vi "Input Quantities.vi"() -> ()   [LabVIEW 2013]
uses:
  qwtblvlib/TD Quantity.ctl
  <vilib>/Analysis/Matrix/Datatypes/RealMatrix.ctl
  globals.vi
  <vilib>/Utility/xml.llb/Write to XML File(string).vi
  <vilib>/Utility/xml.llb/Read From XML File(string).vi
  <vilib>/Utility/file.llb/Read From Spreadsheet File (DBL).vi
  <vilib>/Analysis/Matrix/Numeric/Conversions/Matrix To Array - RM.vi
  <vilib>/Analysis/Matrix/NI_Matrix.lvlib
  qwtblvlib/QWTBLVLib.lvlib
panel:
  out "current Q index":i32 min=0
  in  "r-randomize":bool
  in  "corr-default":bool
  in  "dof-fill":bool
  in  "uncertainty-fill":bool
  in  "value-load CSV":bool
  in  "hide this panel":bool
  in  "load 2clmn csv":bool
  in  "generate wvfrm":bool
  in  "Q changed signal":bool
  in  "reload Q list signal":bool
  in  "reload Q signal":bool
  in  "Q":T1={"Name"="", "Value"=[[1.0]], "Uncertainty"=[[1.0]], "Degrees of Freedom"=[[10.0]], "Correlation"=[[10.0]], "Randomized uncertainty"=[[10.0]]} caption="Selected Quantity"
  in  "load Q":bool
  in  "save Q":bool
  in  "Q list":i32(listbox) caption="List of\nInput Quantities"
  in  "remove Q":bool
  in  "add Q":bool
  in  "rand-clear":bool
  in  "corr-clear":bool
  in  "dof-clear":bool
  in  "uncertainty-clear":bool
  in  "value-clear":bool
  # "Input Quantities"
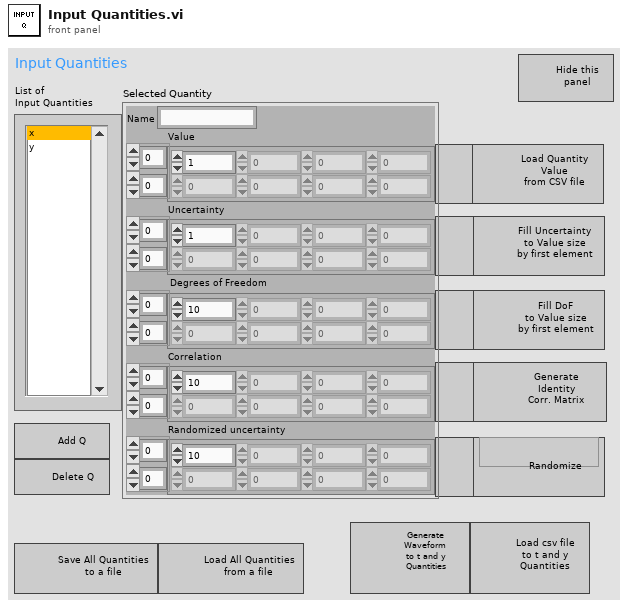
[diagram p1: front panel]
types:
  T1 = typedef "QWTBLVLib.lvlib/TD Quantity.ctl" = cluster{"Name":string, "Value":dbl[][], "Uncertainty":dbl[][], "Degrees of Freedom":dbl[][], "Correlation":dbl[][], "Randomized uncertainty":dbl[][]}
  T2 = enum32{"Invalid", "Standard", "Closed", "Hidden", "Minimized", "Maximized"}
  T3 = cluster{"Name":string, "Value":dbl[][], "Uncertainty":dbl[][], "Degrees of\nFreedom":dbl[][], "Correlation":dbl[][], "Randomized uncertainty":dbl[][]}
  T4 = typedef "NI_Matrix.lvlib/RealMatrix.ctl" = dbl[][]
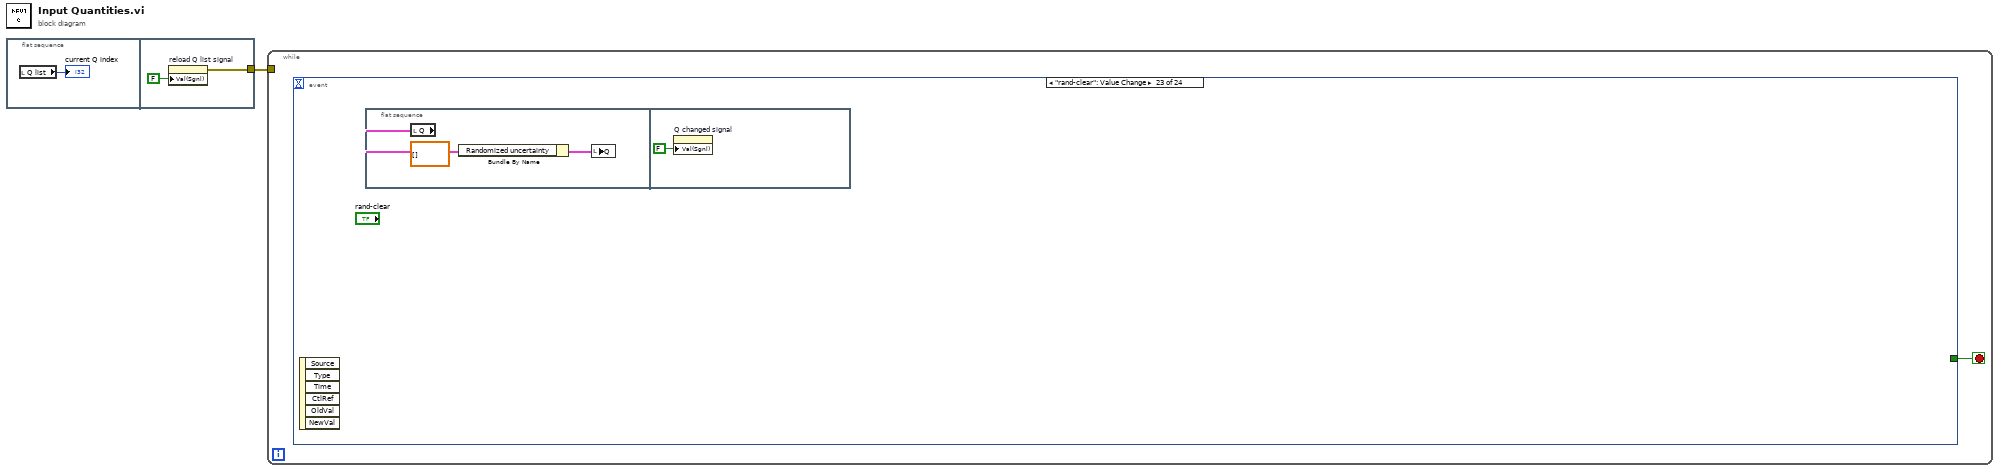
[diagram p0: block diagram]
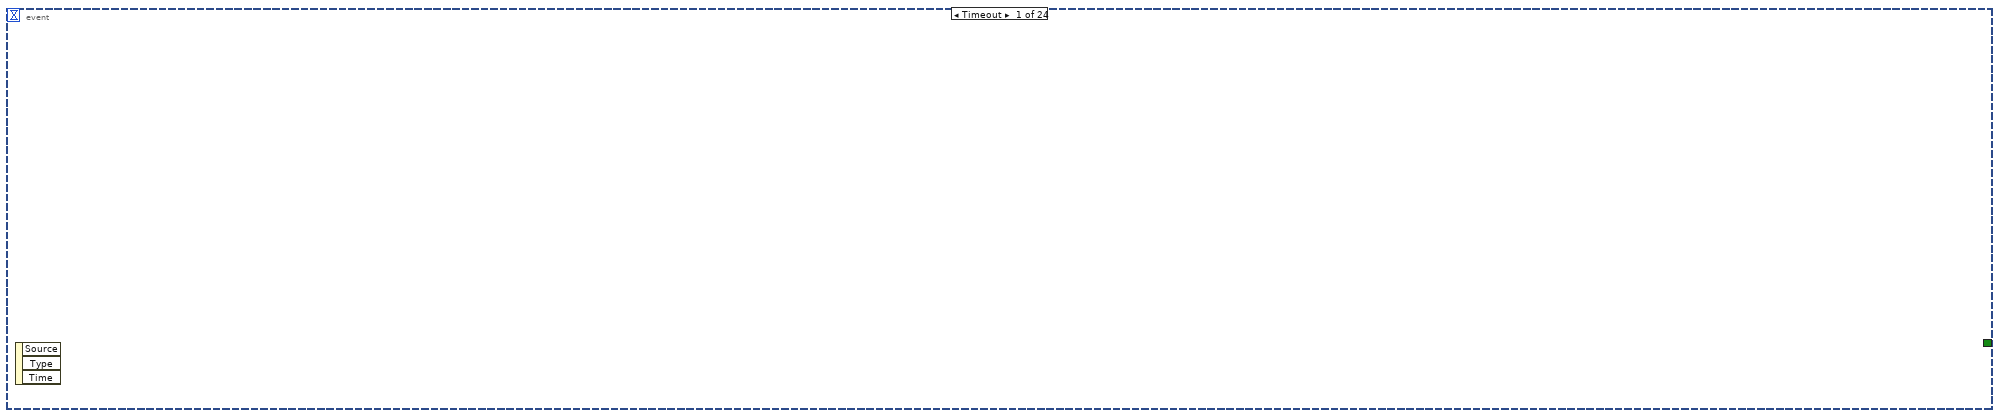
[diagram p2: hidden frame]
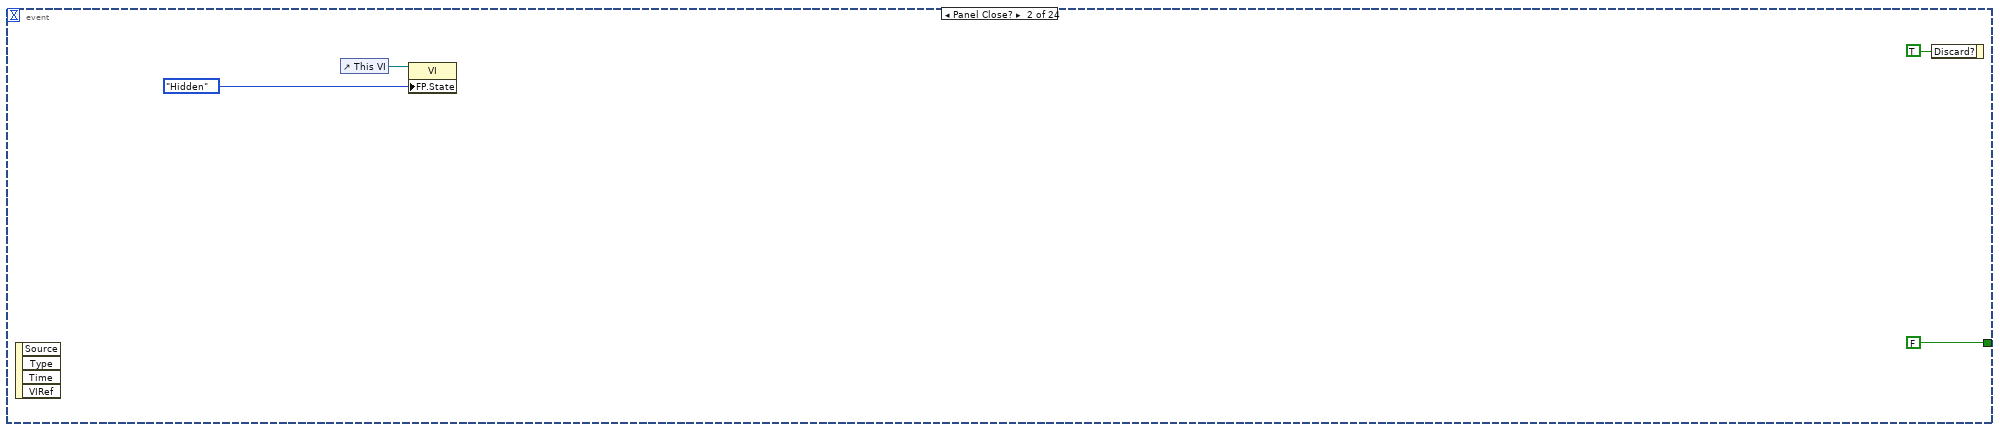
[diagram p3: hidden frame]
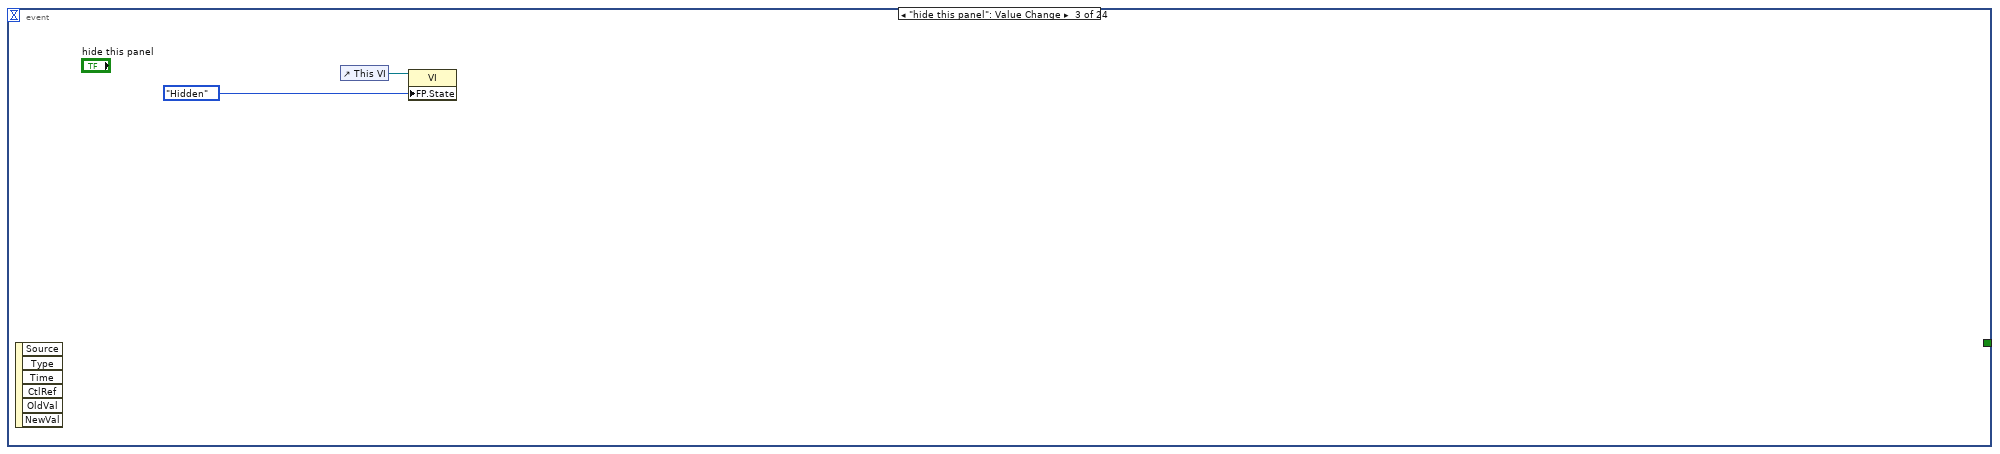
[diagram p4: hidden frame]
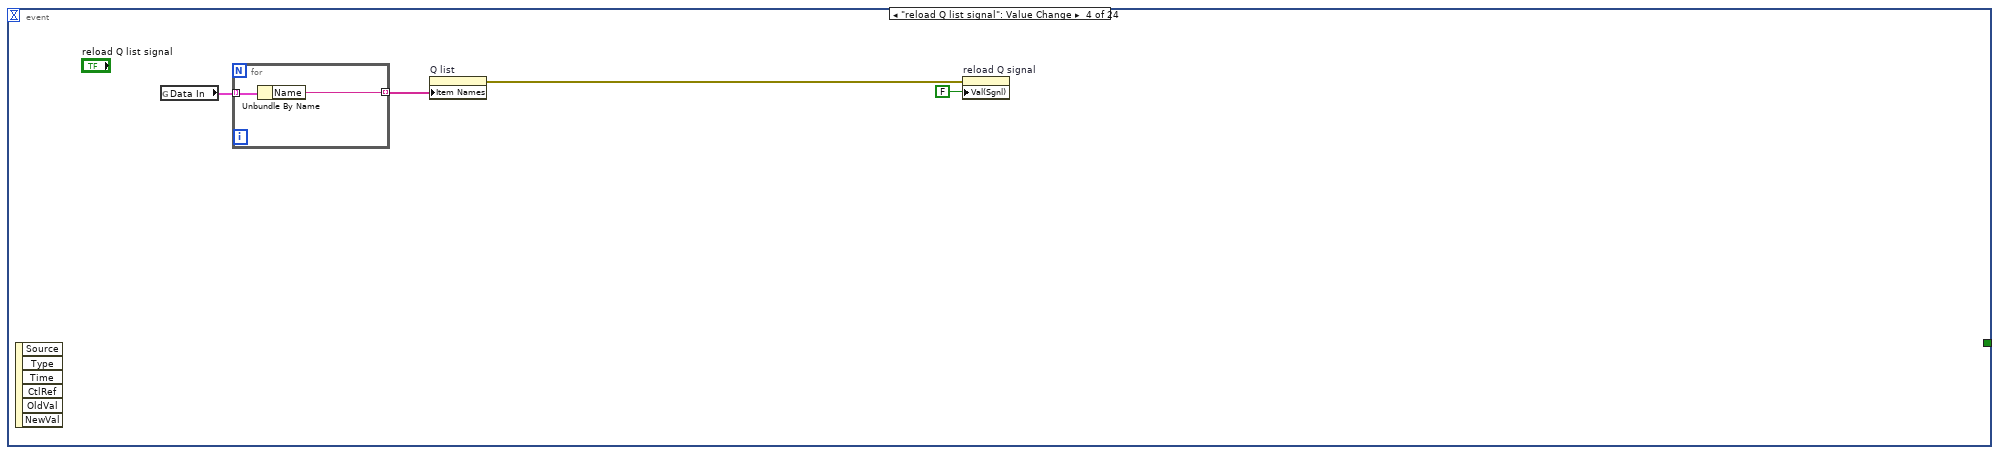
[diagram p5: hidden frame]
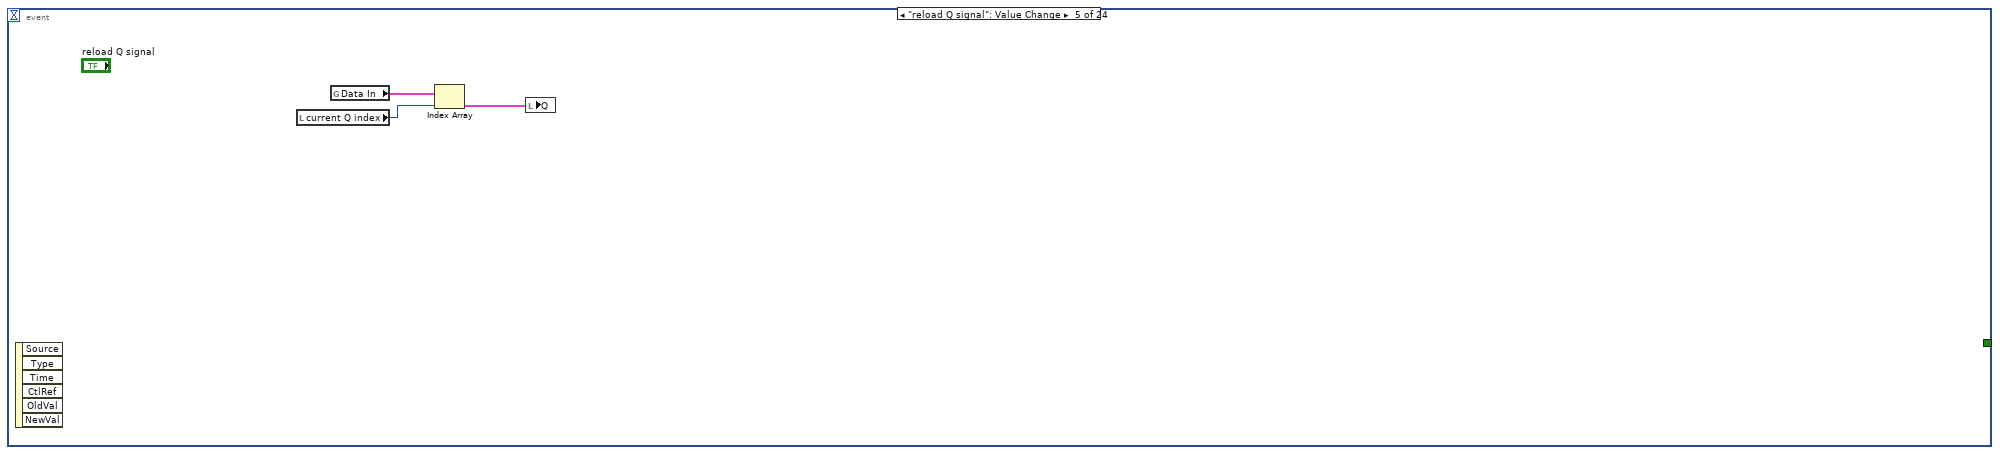
[diagram p6: hidden frame]
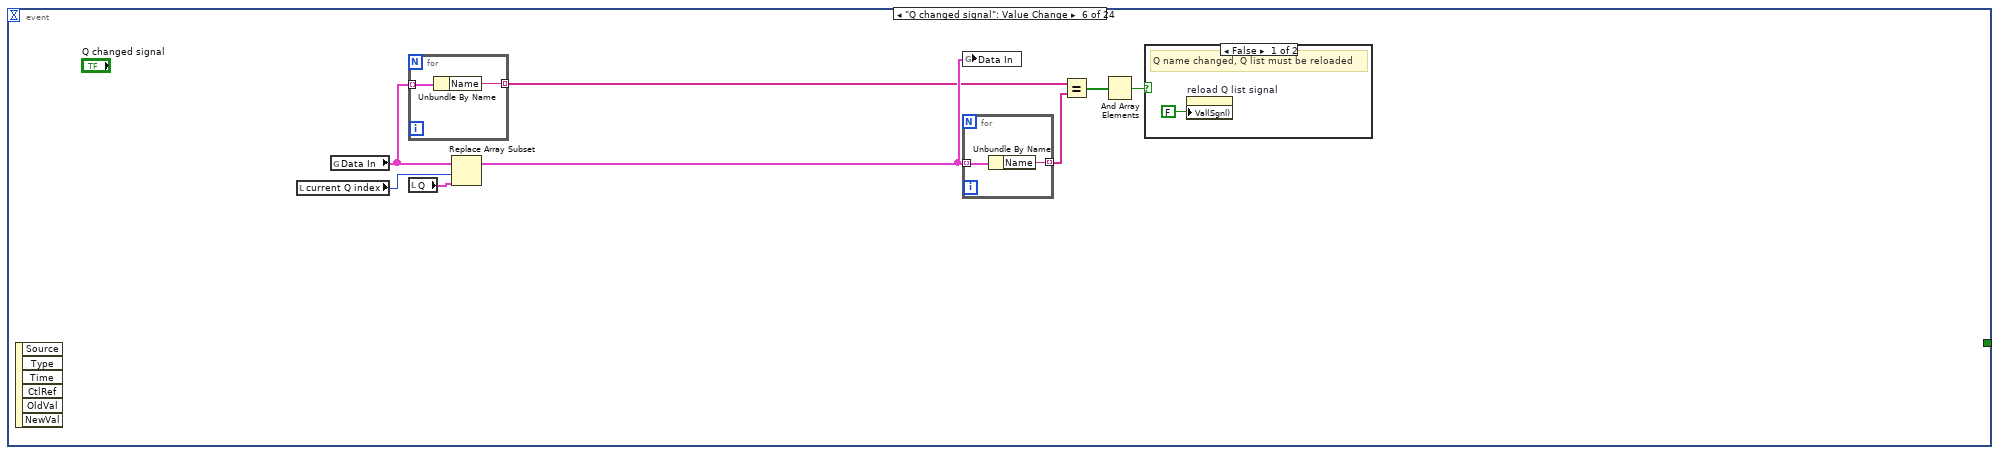
[diagram p7: hidden frame]
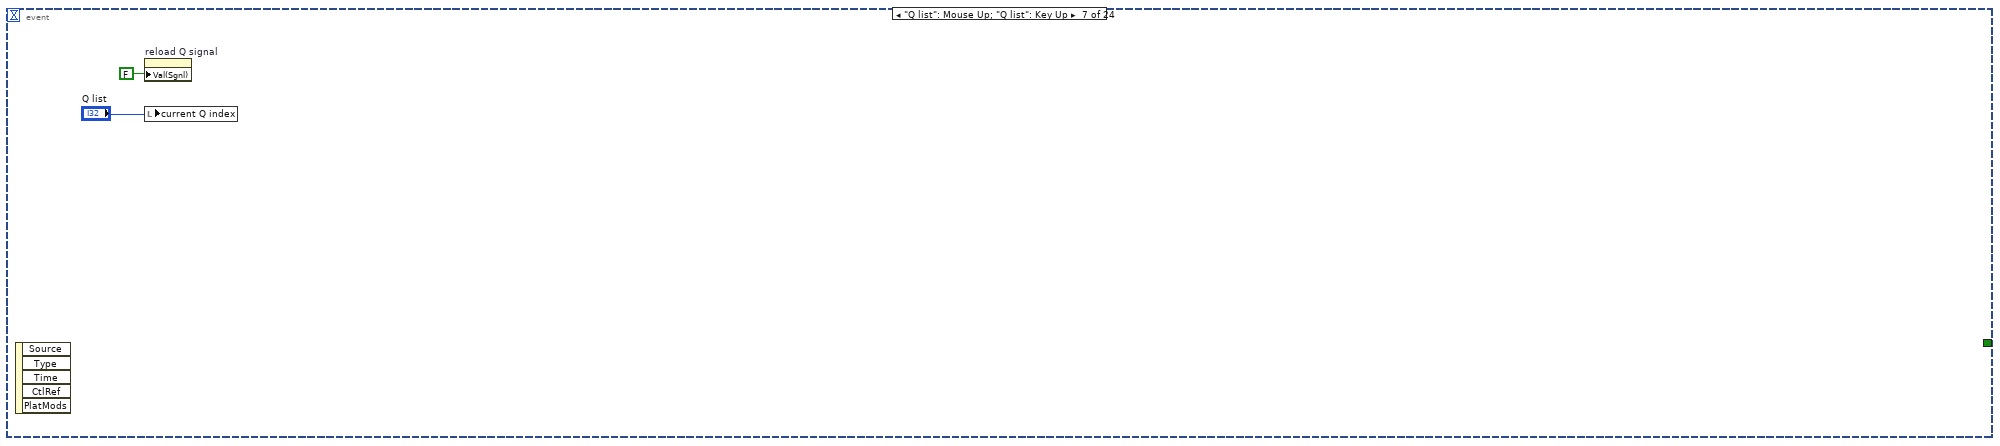
[diagram p9: hidden frame]
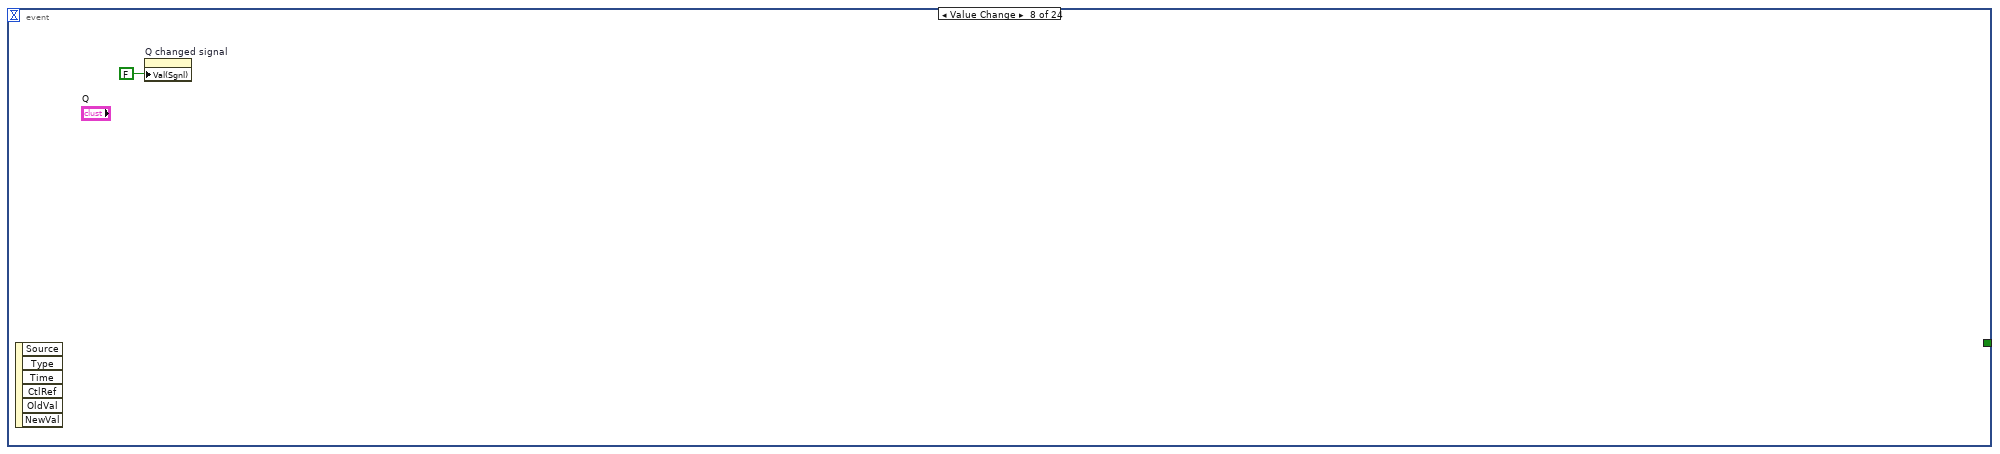
[diagram p10: hidden frame]
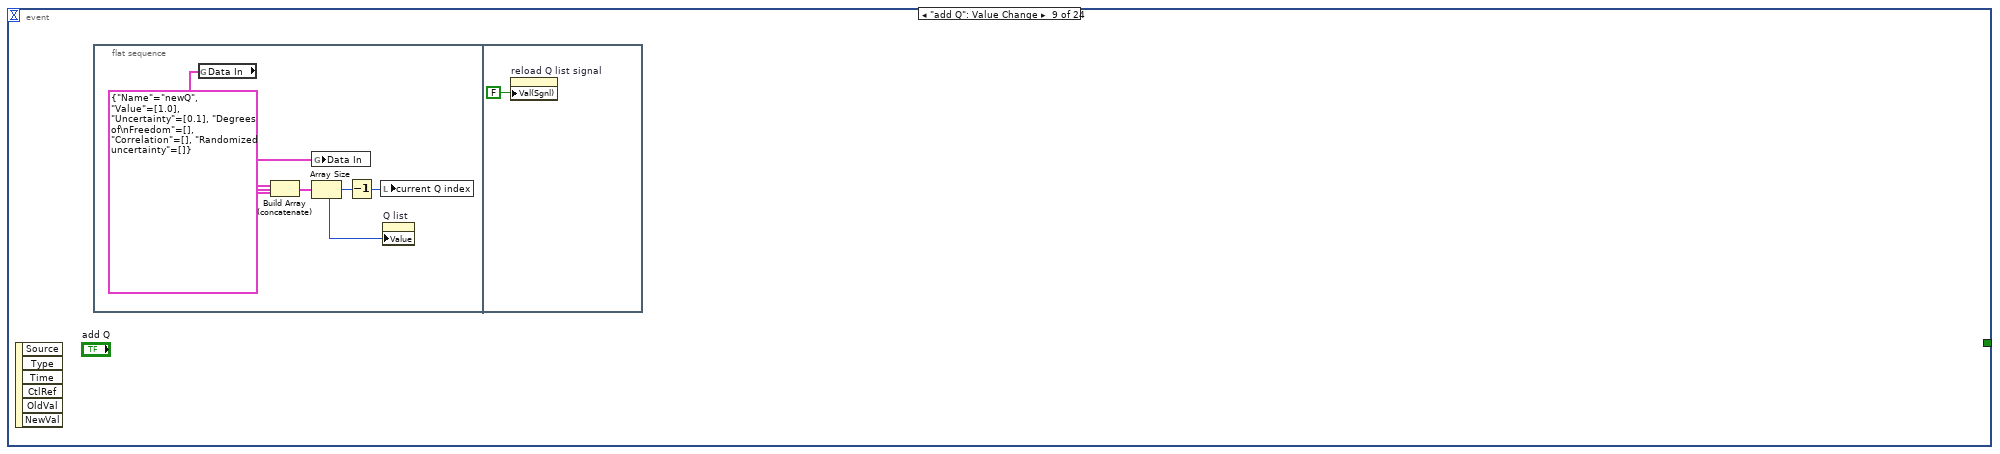
[diagram p11: hidden frame]
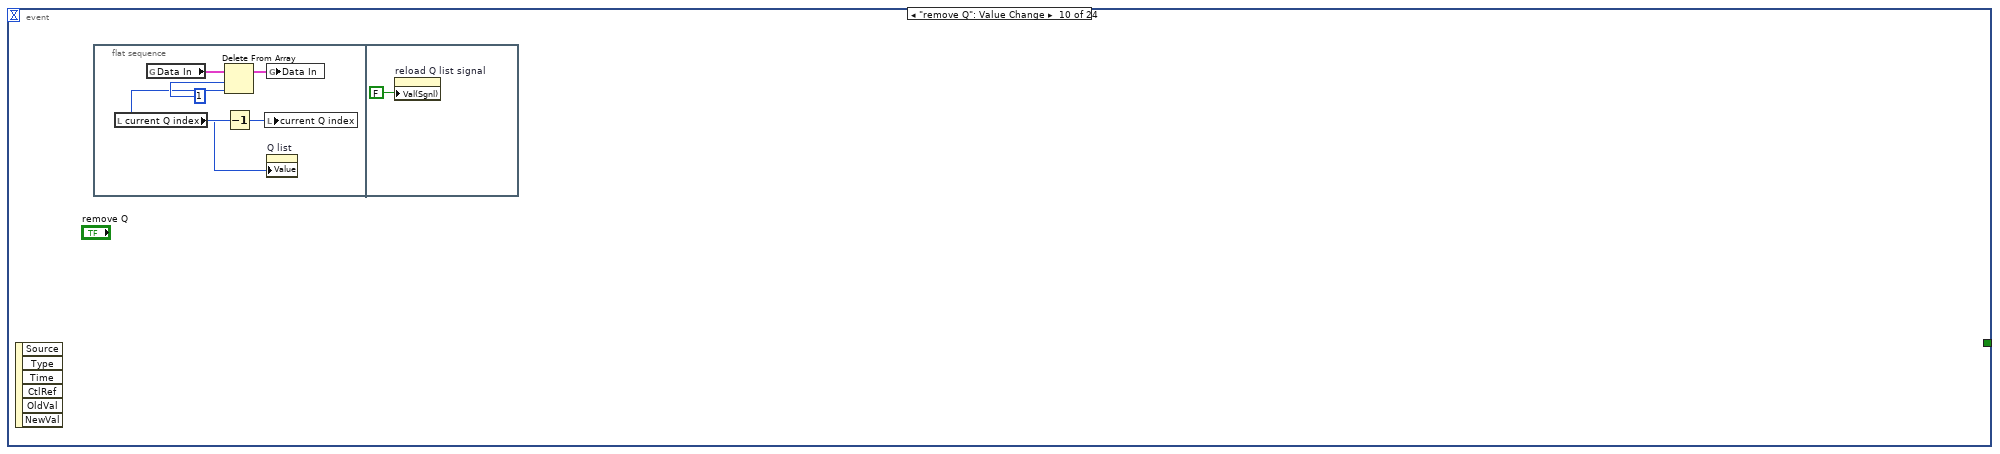
[diagram p12: hidden frame]
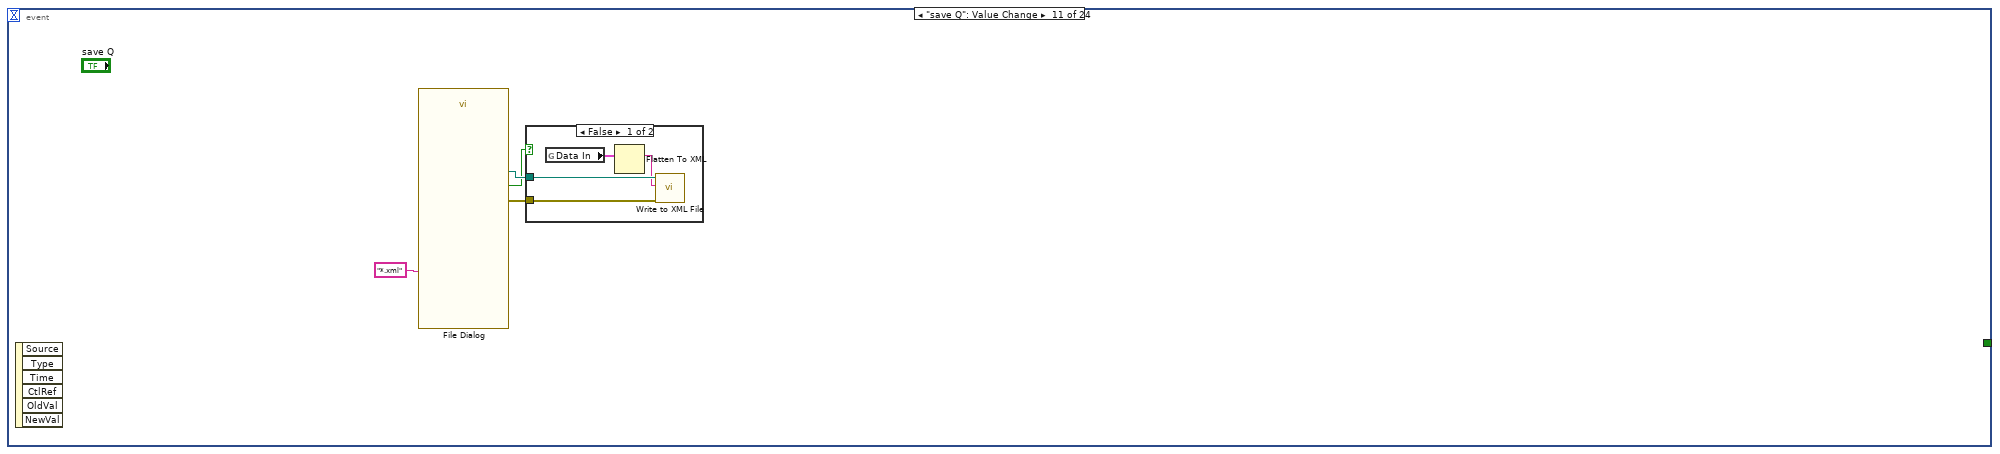
[diagram p13: hidden frame]
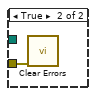
[diagram p14: hidden frame]
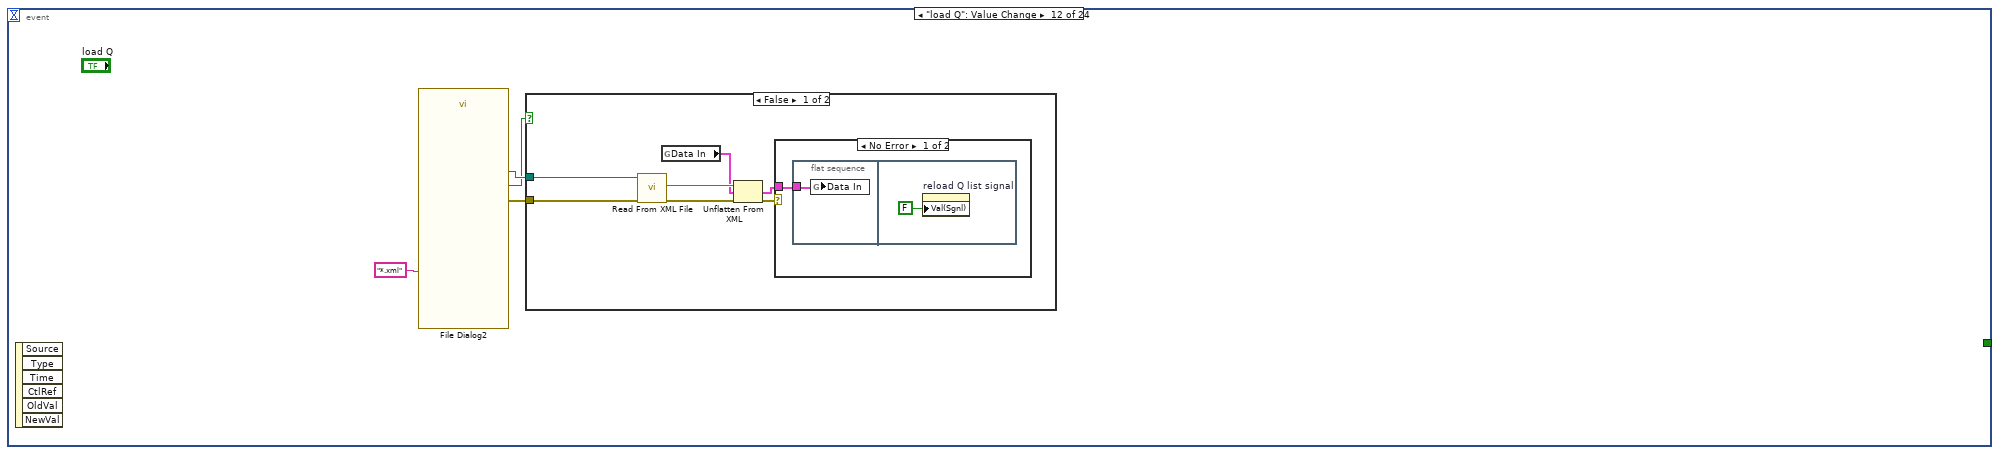
[diagram p15: hidden frame]
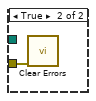
[diagram p17: hidden frame]
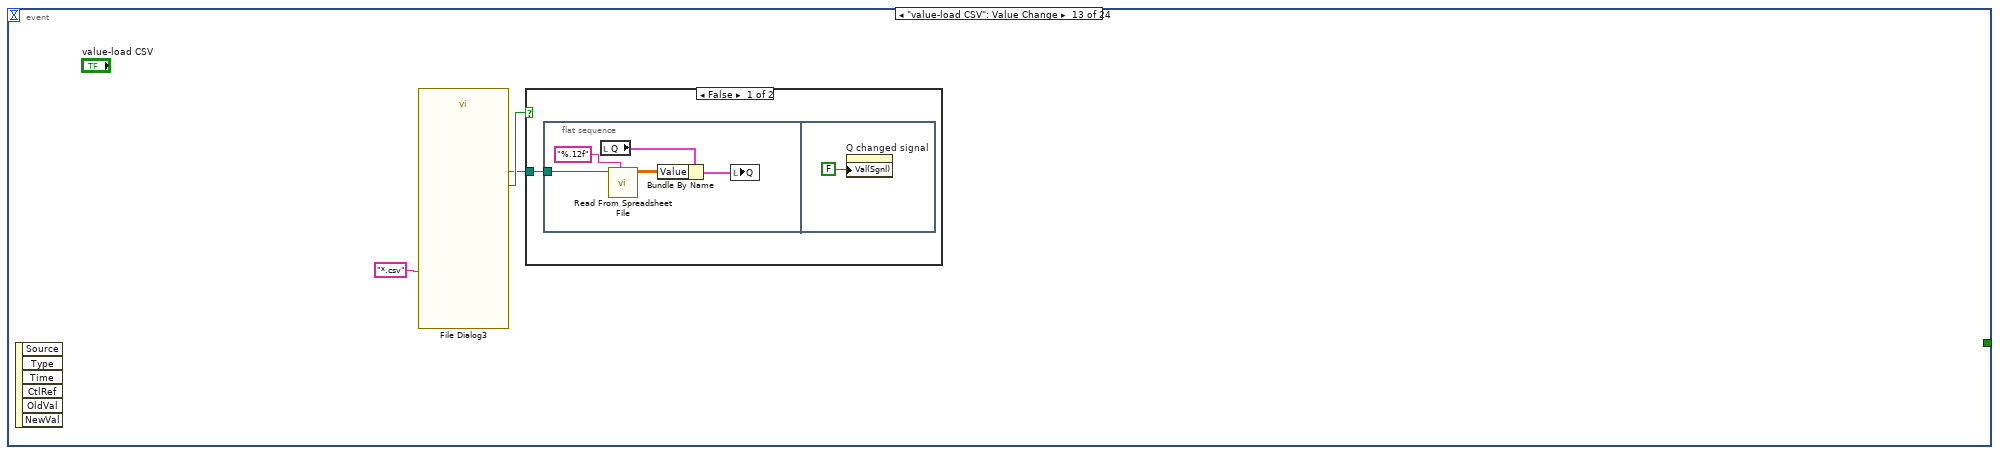
[diagram p18: hidden frame]
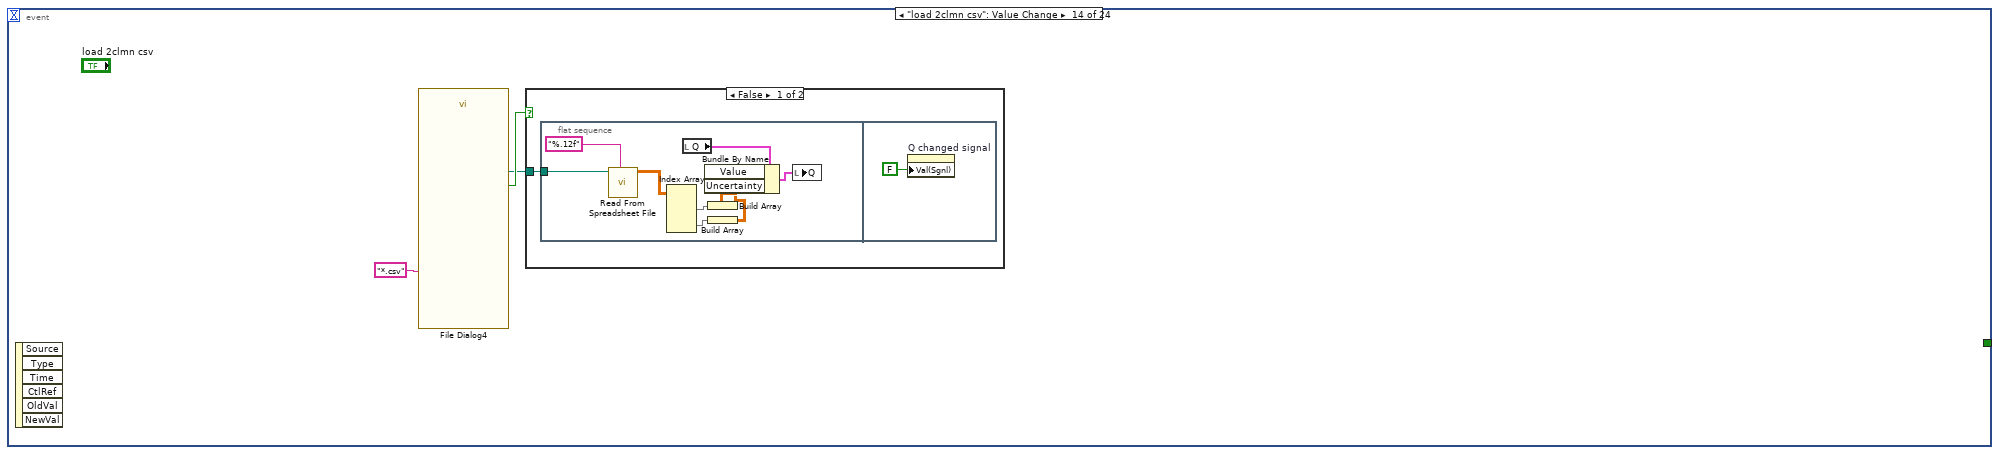
[diagram p20: hidden frame]
diagram:
  n1 = flat-sequence {
    tunnel: [w3] -> w1
    frame #0 {
      n2 = local read "Q list"() -> (→"current Q index":i32)
    }
    frame #1 {
      n3 = property on="reload Q list signal" class="Bool (strict)"("Val(Sgnl)"=FALSE ("Value (Signaling)")) -> (error out=w3:errorcluster)  [unwired: 2 in, 1 out]
    }
  }
  n4 = while {
    tunnel: w1 -> [_]
    stop <- w5 stop-if-true
    n5 = event shown="[22] \"rand-clear\": Value Change" {
      selector: _ -> [_ _ _ _ _ _ _ _ _ _ _ _ _ _ _ _ _ _ _ _ _ _ _ _]
      dyn-events: _ -> [_ _ _ _ _ _ _ _ _ _ _ _ _ _ _ _ _ _ _ _ _ _ _ _]
      timeout: _ -> [_ _ _ _ _ _ _ _ _ _ _ _ _ _ _ _ _ _ _ _ _ _ _ _]
      tunnel: [_ FALSE _ _ _ _ _ _ _ _ _ _ _ _ _ _ _ _ _ _ _ _ _ _] -> w5
      event Timeout {
        n6 = event-data() -> ()  [unwired: 1 in, 3 out]
      }
      event Panel Close? {
        n7 = event-data() -> ()  [unwired: 1 in, 4 out]
        n8 = control-ref of="This VI"() -> (w7:refnum<vi>)
        n9 = property class="VI"(reference=w7, "FP.State"=T2."Hidden" ("Front Panel Window:State")) -> ()  [unwired: 1 in, 2 out]
        n10 = event-data("Discard?"=TRUE) -> ()  [unwired: 1 in, 1 out]
      }
      event "hide this panel": Value Change {
        n11 = event-data() -> ()  [unwired: 1 in, 6 out]
        n12 = control-ref of="This VI"() -> (w11:refnum<vi>)
        n13 = property class="VI"(reference=w11, "FP.State"=T2."Hidden" ("Front Panel Window:State")) -> ()  [unwired: 1 in, 2 out]
      }
      event "reload Q list signal": Value Change {
        n14 = event-data() -> ()  [unwired: 1 in, 6 out]
        n15 = global read "globals.vi" "Data In"() -> (w14:T1[])
        n16 = for {
          tunnel: [w17] -> w13 mode=indexing
          tunnel: w14 -> [w16] mode=indexing
          n17 = Unbundle By Name(w16) -> ("Name"=w17:string)
        }
        n18 = property on="Q list" class="LstBox (strict)"("Item Names"=w13) -> (error out=w12:errorcluster)  [unwired: 2 in, 1 out]
        n19 = property on="reload Q signal" class="Bool (strict)"(error in=w12, "Val(Sgnl)"=FALSE ("Value (Signaling)")) -> ()  [unwired: 1 in, 2 out]
      }
      event "reload Q signal": Value Change {
        n20 = event-data() -> ()  [unwired: 1 in, 6 out]
        n21 = local read "current Q index"() -> (w18:i32)
        n22 = global read "globals.vi" "Data In"() -> (w20:T1[])
        n23 = Index Array(array=w20, index=w18) -> (element=w19:T1)
        n24 = local write "Q"(w19) -> ()
      }
      event "Q changed signal": Value Change {
        n25 = event-data() -> ()  [unwired: 1 in, 6 out]
        n26 = local read "current Q index"() -> (w21:i32)
        n27 = global read "globals.vi" "Data In"() -> (w27:T1[])
        n28 = for {
          tunnel: [w32] -> w25 mode=indexing
          tunnel: w27 -> [w31] mode=indexing
          n29 = Unbundle By Name(w31) -> ("Name"=w32:string)
        }
        n30 = local read "Q"() -> (w28:T1)
        n31 = Replace Array Subset(array=w27, new element=w28, index=w21) -> (w26:T1[])
        n32 = global write "globals.vi" "Data In"(w26) -> ()
        n33 = for {
          tunnel: [w30] -> w23 mode=indexing
          tunnel: w26 -> [w29] mode=indexing
          n34 = Unbundle By Name(w29) -> ("Name"=w30:string)
        }
        n35 = Equal?(x=w25, y=w23) -> (x = y?=w22:bool[])
        n36 = And Array Elements(Boolean array=w22) -> (logical AND=w24:bool)
        n37 = case shown="False" w24 {
          frame False {
            # "Q name changed, Q list must be reloaded"
            n38 = property on="reload Q list signal" class="Bool (strict)"("Val(Sgnl)"=FALSE ("Value (Signaling)")) -> ()  [unwired: 2 in, 2 out]
          }
          frame True {
          }
        }
      }
      event "Q list": Mouse Up; "Q list": Key Up {
        n39 = event-data() -> ()  [unwired: 1 in, 5 out]
        n40 = property on="reload Q signal" class="Bool (strict)"("Val(Sgnl)"=FALSE ("Value (Signaling)")) -> ()  [unwired: 2 in, 2 out]
        n41 = local write "current Q index"("Q list") -> ()
      }
      event Value Change {
        n42 = event-data() -> ()  [unwired: 1 in, 6 out]
        n43 = property on="Q changed signal" class="Bool (strict)"("Val(Sgnl)"=FALSE ("Value (Signaling)")) -> ()  [unwired: 2 in, 2 out]
      }
      event "add Q": Value Change {
        n44 = event-data() -> ()  [unwired: 1 in, 6 out]
        n45 = flat-sequence {
          frame #0 {
            n46 = global read "globals.vi" "Data In"() -> (w39:T1[])
            n47 = Build Array (concatenate)(w39, T3 {"Name"="newQ", "Value"=[[1.0]], "Uncertainty"=[[0.1]], "Degrees of\nFreedom"=[], "Correlation"=[], "Randomized uncertainty"=[]} ("Quantity")) -> (w38:T1[])
            n48 = global write "globals.vi" "Data In"(w38) -> ()
            n49 = Array Size(array=w38) -> (size(s)=w41:i32)
            n50 = Decrement(x=w41) -> (x-1=w37:i32)
            n51 = local write "current Q index"(w37) -> ()
            n52 = property on="Q list" class="LstBox (strict)"("Value"=w37) -> ()  [unwired: 2 in, 2 out]
          }
          frame #1 {
            n53 = property on="reload Q list signal" class="Bool (strict)"("Val(Sgnl)"=FALSE ("Value (Signaling)")) -> ()  [unwired: 2 in, 2 out]
          }
        }
      }
      event "remove Q": Value Change {
        n54 = event-data() -> ()  [unwired: 1 in, 6 out]
        n55 = flat-sequence {
          frame #0 {
            n56 = local read "current Q index"() -> (w44:i32)
            n57 = global read "globals.vi" "Data In"() -> (w46:T1[])
            n58 = Delete From Array(array=w46, length=1, index=w44) -> (array with subset deleted=w45:T1[])  [unwired: 1 out]
            n59 = Decrement(x=w44) -> (x-1=w43:i32)
            n60 = local write "current Q index"(w43) -> ()
            n61 = global write "globals.vi" "Data In"(w45) -> ()
            n62 = property on="Q list" class="LstBox (strict)"("Value"=w43) -> ()  [unwired: 2 in, 2 out]
          }
          frame #1 {
            n63 = property on="reload Q list signal" class="Bool (strict)"("Val(Sgnl)"=FALSE ("Value (Signaling)")) -> ()  [unwired: 2 in, 2 out]
          }
        }
      }
      event "save Q": Value Change {
        n64 = event-data() -> ()  [unwired: 1 in, 6 out]
        n65 = call "File Dialog"("pattern (all files)"="*.xml") -> ("selected path"=w52:path, "cancelled"=w50:bool, "error out"=w51:errorcluster)  [unwired: 11 in, 1 out]
        n66 = case shown="False" w50 {
          tunnel: w51 -> [w55 w57]
          tunnel: w52 -> [w56 _]
          frame False {
            n67 = global read "globals.vi" "Data In"() -> (w53:T1[])
            n68 = Flatten To XML(anything=w53) -> (xml string=w54:string)
            n69 = call-poly <vilib>:"Write to XML File.vi"("error in (no error)"=w55, "XML Input"=w54, "XML File Path"=w56) -> ()  [unwired: 6 in, 3 out]
          }
          frame True {
            n70 = call <vilib>:"Clear Errors.vi"("error in (no error)"=w57) -> ()  [unwired: 6 in, 1 out]
          }
        }
      }
      event "load Q": Value Change {
        n71 = event-data() -> ()  [unwired: 1 in, 6 out]
        n72 = call "File Dialog2"("pattern (all files)"="*.xml") -> ("selected path"=w61:path, "cancelled"=w59:bool, "error out"=w60:errorcluster)  [unwired: 11 in, 1 out]
        n73 = case shown="False" w59 {
          tunnel: w60 -> [w67 w72]
          tunnel: w61 -> [w68 _]
          frame False {
            n74 = call-poly <vilib>:"Read From XML File.vi"("error in (no error)"=w67, "XML File Path"=w68) -> ("error out"=w65:errorcluster, "XML Elements"=w66:string)  [unwired: 7 in, 1 out]
            n75 = global read "globals.vi" "Data In"() -> (w62:T1[])
            n76 = Unflatten From XML(xml string=w66, type=w62, error in (no error)=w65) -> (value=w63:T1[], error out=w64:errorcluster)
            n77 = case shown="No Error" w64 {
              tunnel: w63 -> [w69 _]
              frame No Error {
                n78 = flat-sequence {
                  tunnel: w69 -> [w70]
                  frame #0 {
                    n79 = global write "globals.vi" "Data In"(w70) -> ()
                  }
                  frame #1 {
                    n80 = property on="reload Q list signal" class="Bool (strict)"("Val(Sgnl)"=FALSE ("Value (Signaling)")) -> ()  [unwired: 2 in, 2 out]
                  }
                }
              }
              frame Error {
              }
            }
          }
          frame True {
            n81 = call <vilib>:"Clear Errors.vi"("error in (no error)"=w72) -> ()  [unwired: 6 in, 1 out]
          }
        }
      }
      event "value-load CSV": Value Change {
        n82 = event-data() -> ()  [unwired: 1 in, 6 out]
        n83 = call "File Dialog3"("pattern (all files)"="*.csv") -> ("selected path"=w73:path, "cancelled"=w74:bool)  [unwired: 11 in, 2 out]
        n84 = case shown="False" w74 {
          tunnel: w73 -> [w76 _]
          frame False {
            n85 = flat-sequence {
              tunnel: w76 -> [w81]
              frame #0 {
                n86 = local read "Q"() -> (w80:T1)
                n87 = call-poly <vilib>:"Read From Spreadsheet File.vi"("format (%.3f)"="%.12f", "file path (dialog if empty)"=w81) -> ("all rows"=w79:dbl[][])  [unwired: 5 in, 4 out]
                n88 = Bundle By Name(cluster=w80, "Value"=w79) -> (w78:T1)
                n89 = local write "Q"(w78) -> ()
              }
              frame #1 {
                n90 = property on="Q changed signal" class="Bool (strict)"("Val(Sgnl)"=FALSE ("Value (Signaling)")) -> ()  [unwired: 2 in, 2 out]
              }
            }
          }
          frame True {
          }
        }
      }
      event "load 2clmn csv": Value Change {
        n91 = event-data() -> ()  [unwired: 1 in, 6 out]
        n92 = call "File Dialog4"("pattern (all files)"="*.csv") -> ("selected path"=w83:path, "cancelled"=w84:bool)  [unwired: 11 in, 2 out]
        n93 = case shown="False" w84 {
          tunnel: w83 -> [w86 _]
          frame False {
            n94 = flat-sequence {
              tunnel: w86 -> [w95]
              frame #0 {
                n95 = call-poly <vilib>:"Read From Spreadsheet File.vi"("format (%.3f)"="%.12f", "file path (dialog if empty)"=w95) -> ("all rows"=w91:dbl[][])  [unwired: 5 in, 4 out]
                n96 = Index Array(array=w91) -> (element #1=w90:dbl[], element #2=w87:dbl[])  [unwired: 4 in]
                n97 = local read "Q"() -> (w94:T1)
                n98 = Build Array(w90) -> (w89:dbl[][])
                n99 = Build Array(w87) -> (w88:dbl[][])
                n100 = Bundle By Name(cluster=w94, "Value"=w89, "Uncertainty"=w88) -> (w93:T1)
                n101 = local write "Q"(w93) -> ()
              }
              frame #1 {
                n102 = property on="Q changed signal" class="Bool (strict)"("Val(Sgnl)"=FALSE ("Value (Signaling)")) -> ()  [unwired: 2 in, 2 out]
              }
            }
          }
          frame True {
          }
        }
      }
      event "uncertainty-fill": Value Change {
        n103 = event-data() -> ()  [unwired: 1 in, 6 out]
        n104 = flat-sequence {
          frame #0 {
            n105 = local read "Q"() -> (w109:T1)
            n106 = Unbundle By Name(w109) -> ("Value"=w107:dbl[][], "Uncertainty"=w97:dbl[][])
            n107 = Array Size(array=w107) -> (size(s)=w103:i32[])
            n108 = Index Array(array=w97, index (row)=0, index (col)=0 ("disabled index (col)")) -> (element=w104:dbl)
            n109 = Index Array(array=w103, index #1=0 ("index"), index #2=1 ("index")) -> (element #1=w100:i32, element #2=w99:i32)
            n110 = Initialize Array(w104, w100, w99) -> (w98:dbl[][])
            n111 = Bundle By Name(cluster=w109, "Uncertainty"=w98) -> (w108:T1)
            n112 = local write "Q"(w108) -> ()
          }
          frame #1 {
            n113 = property on="Q changed signal" class="Bool (strict)"("Val(Sgnl)"=FALSE ("Value (Signaling)")) -> ()  [unwired: 2 in, 2 out]
          }
        }
      }
      event "dof-fill": Value Change {
        n114 = event-data() -> ()  [unwired: 1 in, 6 out]
        n115 = flat-sequence {
          frame #0 {
            n116 = local read "Q"() -> (w123:T1)
            n117 = Unbundle By Name(w123) -> ("Value"=w121:dbl[][], "Degrees of Freedom"=w111:dbl[][])
            n118 = Array Size(array=w121) -> (size(s)=w117:i32[])
            n119 = Index Array(array=w111, index (row)=0, index (col)=0 ("disabled index (col)")) -> (element=w118:dbl)
            n120 = Index Array(array=w117, index #1=0 ("index"), index #2=1 ("index")) -> (element #1=w114:i32, element #2=w113:i32)
            n121 = Initialize Array(w118, w114, w113) -> (w112:dbl[][])
            n122 = Bundle By Name(cluster=w123, "Degrees of Freedom"=w112) -> (w122:T1)
            n123 = local write "Q"(w122) -> ()
          }
          frame #1 {
            n124 = property on="Q changed signal" class="Bool (strict)"("Val(Sgnl)"=FALSE ("Value (Signaling)")) -> ()  [unwired: 2 in, 2 out]
          }
        }
      }
      event "corr-default": Value Change {
        n125 = event-data() -> ()  [unwired: 1 in, 6 out]
        n126 = flat-sequence {
          frame #0 {
            n127 = local read "Q"() -> (w131:T1)
            n128 = Unbundle By Name(w131) -> ("Value"=w129:dbl[][])
            n129 = call "Scalar Vector Matrix in 2D.vi"("2D Array"=w129) -> ("Is Matrix?"=w128:bool, "Is Empty?"=w125:bool, "Dim Max"=w126:i32, "Dimensions"=w127:i32[])  [unwired: 4 in, 3 out]
            n130 = case shown="True" w125 {
              tunnel: w131 -> [w136 w150]
              tunnel: [w135 w149] -> w130
              tunnel: w128 -> [w134 _]
              tunnel: w127 -> [w133 _]
              tunnel: w126 -> [w132 _]
              frame False {
                # "vector or matrix"
                n131 = case shown="False" w134 {
                  tunnel: w136 -> [w146 w147]
                  tunnel: [w145 w147] -> w135
                  tunnel: w133 -> [_ _]
                  tunnel: w132 -> [w137 _]
                  frame False {
                    # "vector"
                    n132 = Resize Matrix(1:w137, 2:w137, 4:T4 [] ("matrix")) -> (0:w140:T4)
                    n133 = Replace Array Subset(array=w140, new element=1.0 ("new diagonal/fill element"), index (row)=0 ("disabled index (row)"), index (col)=0 ("disabled index (col)")) -> (w139:T4)
                    n134 = call-poly <vilib>:"Matrix To Array.vi"("Real Matrix"=w139) -> ("Real 2D Array"=w138:dbl[][])
                    n135 = Bundle By Name(cluster=w146, "Correlation"=w138) -> (w145:T1)
                  }
                  frame True {
                    # "matrix"
                  }
                }
              }
              frame True {
                # "empty array"
                n136 = Bundle By Name(cluster=w150, "Correlation"=dbl[][] []) -> (w149:T1)
              }
            }
            n137 = local write "Q"(w130) -> ()
          }
          frame #1 {
            n138 = property on="Q changed signal" class="Bool (strict)"("Val(Sgnl)"=FALSE ("Value (Signaling)")) -> ()  [unwired: 2 in, 2 out]
          }
        }
      }
      event "r-randomize": Value Change {
        # "#2do"
        n139 = event-data() -> ()  [unwired: 1 in, 6 out]
        n140 = local read "Q"() -> (w158:T1)
        n141 = Unbundle By Name(w158) -> ("Value"=w162:dbl[][], "Uncertainty"=w156:dbl[][])
        n142 = call "Scalar Vector Matrix in 2D.vi"("2D Array"=w162) -> ("Is Matrix?"=w161:bool, "Is Vector?"=w157:bool, "Is Empty?"=w159:bool, "Dim Max"=w155:i32, "Dim Min"=w154:i32)  [unwired: 4 in, 2 out]
        n143 = Or(x=w159, y=w161) -> (x .or. y?=w160:bool)
        n144 = case shown="False" w160 {
          tunnel: w159 -> [_ w185]
          tunnel: w158 -> [w176 w184]
          tunnel: w157 -> [_ _]
          tunnel: w156 -> [w175 _]
          tunnel: w155 -> [w174 _]
          tunnel: w154 -> [w172 _]
          tunnel: [w167 w184] -> w153
          tunnel: [w166 TRUE ("Canceled?")] -> w152
          frame False {
            n145 = call "Scalar Vector Matrix in 2D.vi"("2D Array"=w175) -> ("Dim Max"=w173:i32, "Dim Min"=w171:i32)  [unwired: 4 in, 5 out]
            n146 = Equal?(x=w174, y=w173) -> (x = y?=w169:bool)
            n147 = Equal?(x=w172, y=w171) -> (x = y?=w170:bool)
            n148 = And(x=w169, y=w170) -> (x .and. y?=w168:bool)
            n149 = case shown="True" w168 {
              tunnel: w176 -> [w178 w182]
              tunnel: [w178 w181] -> w167
              tunnel: [TRUE ("Canceled?") w180] -> w166
              frame False {
                n150 = One Button Dialog(message="Values and uncertainties of Quantity\nhas different dimensions.") -> ()  [unwired: 1 in, 1 out]
              }
              frame True {
                n151 = call "Randomize.vi"("Quantity"=w182) -> ("Canceled?"=w180:bool, "Randomized Quantity"=w181:T1)  [unwired: 9 in]
              }
            }
          }
          frame True {
            n152 = case shown="False" w185 {
              frame False {
                n153 = One Button Dialog(message="Cannot do for matrix quantity.\nImplemented only for scalars or vectors.", button name ("OK")="OK") -> ()  [unwired: 1 out]
              }
              frame True {
                n154 = One Button Dialog(message="Value matrix is empty!", button name ("OK")="OK") -> ()  [unwired: 1 out]
              }
            }
          }
        }
        n155 = case shown="False" w152 {
          tunnel: w153 -> [w163 _]
          frame False {
            n156 = flat-sequence {
              tunnel: w163 -> [w164]
              frame #0 {
                n157 = local write "Q"(w164) -> ()
              }
              frame #1 {
                n158 = property on="Q changed signal" class="Bool (strict)"("Val(Sgnl)"=FALSE ("Value (Signaling)")) -> ()  [unwired: 2 in, 2 out]
              }
            }
          }
          frame True {
          }
        }
      }
      event "value-clear": Value Change {
        n159 = event-data() -> ()  [unwired: 1 in, 6 out]
        n160 = flat-sequence {
          frame #0 {
            n161 = local read "Q"() -> (w192:T1)
            n162 = Bundle By Name(cluster=w192, "Value"=dbl[][] []) -> (w191:T1)
            n163 = local write "Q"(w191) -> ()
          }
          frame #1 {
            n164 = property on="Q changed signal" class="Bool (strict)"("Val(Sgnl)"=FALSE ("Value (Signaling)")) -> ()  [unwired: 2 in, 2 out]
          }
        }
      }
      event "uncertainty-clear": Value Change {
        n165 = event-data() -> ()  [unwired: 1 in, 6 out]
        n166 = flat-sequence {
          frame #0 {
            n167 = local read "Q"() -> (w196:T1)
            n168 = Bundle By Name(cluster=w196, "Uncertainty"=dbl[][] [] ("Value")) -> (w195:T1)
            n169 = local write "Q"(w195) -> ()
          }
          frame #1 {
            n170 = property on="Q changed signal" class="Bool (strict)"("Val(Sgnl)"=FALSE ("Value (Signaling)")) -> ()  [unwired: 2 in, 2 out]
          }
        }
      }
      event "dof-clear": Value Change {
        n171 = event-data() -> ()  [unwired: 1 in, 6 out]
        n172 = flat-sequence {
          frame #0 {
            n173 = local read "Q"() -> (w200:T1)
            n174 = Bundle By Name(cluster=w200, "Degrees of Freedom"=dbl[][] [] ("Value")) -> (w199:T1)
            n175 = local write "Q"(w199) -> ()
          }
          frame #1 {
            n176 = property on="Q changed signal" class="Bool (strict)"("Val(Sgnl)"=FALSE ("Value (Signaling)")) -> ()  [unwired: 2 in, 2 out]
          }
        }
      }
      event "corr-clear": Value Change {
        n177 = event-data() -> ()  [unwired: 1 in, 6 out]
        n178 = flat-sequence {
          frame #0 {
            n179 = local read "Q"() -> (w204:T1)
            n180 = Bundle By Name(cluster=w204, "Correlation"=dbl[][] [] ("Value")) -> (w203:T1)
            n181 = local write "Q"(w203) -> ()
          }
          frame #1 {
            n182 = property on="Q changed signal" class="Bool (strict)"("Val(Sgnl)"=FALSE ("Value (Signaling)")) -> ()  [unwired: 2 in, 2 out]
          }
        }
      }
      event "rand-clear": Value Change {
        n183 = event-data() -> ()  [unwired: 1 in, 6 out]
        n184 = flat-sequence {
          frame #0 {
            n185 = local read "Q"() -> (w208:T1)
            n186 = Bundle By Name(cluster=w208, "Randomized uncertainty"=dbl[][] [] ("Value")) -> (w207:T1)
            n187 = local write "Q"(w207) -> ()
          }
          frame #1 {
            n188 = property on="Q changed signal" class="Bool (strict)"("Val(Sgnl)"=FALSE ("Value (Signaling)")) -> ()  [unwired: 2 in, 2 out]
          }
        }
      }
      event "generate wvfrm": Value Change {
        n189 = event-data() -> ()  [unwired: 1 in, 6 out]
        n190 = call "generate wvfrm.vi"() -> ("error out"=w212:errorcluster, "waveform"=w210:dbl[], "time series"=w211:dbl[], "canceled?"=w213:bool)  [unwired: 8 in]
        n191 = case shown="False" w213 {
          tunnel: w212 -> [w216 _]
          tunnel: w211 -> [w215 _]
          tunnel: w210 -> [w214 _]
          frame False {
            # "not canceled"
            n192 = case shown="No Error" w216 {
              tunnel: w215 -> [w225 _]
              tunnel: w214 -> [w221 _]
              frame No Error {
                w219 = T3 {"Name"="", "Value"=[], "Uncertainty"=[], "Degrees of\nFreedom"=[], "Correlation"=[], "Randomized uncertainty"=[]} ("Quantity")
                n193 = Build Array(w225) -> (w224:dbl[][])
                n194 = Build Array(w221) -> (w220:dbl[][])
                n195 = global read "globals.vi" "Data In"() -> (w229:T1[])
                n196 = Bundle By Name(cluster=w219, "Name"="t", "Value"=w224) -> (w217:T3)
                n197 = Bundle By Name(cluster=w219, "Name"="y", "Value"=w220) -> (w218:T3)
                n198 = Build Array (concatenate)(w229, w217, w218) -> (w226:T1[])
                n199 = global write "globals.vi" "Data In"(w226) -> ()
                n200 = Array Size(array=w226) -> (size(s)=w231:i32)
                n201 = Decrement(x=w231) -> (x-1=w230:i32)
                n202 = property on="Q list" class="LstBox (strict)"("Value"=w230) -> (error out=w227:errorcluster)  [unwired: 2 in, 1 out]
                n203 = property on="reload Q list signal" class="Bool (strict)"(error in=w227, "Val(Sgnl)"=FALSE ("Value (Signaling)")) -> ()  [unwired: 1 in, 2 out]
              }
              frame Error {
              }
            }
          }
          frame True {
          }
        }
      }
    }
  }
